vi "Encode.vi"(4 "Conf":T1, 5 "Controller 2 State":T2={"Left X"=0, "Left Y"=0, "Right X"=0, "Right Y"=0, "Button Encoding 9-12"=0, "Button Encoding 1-8"=0, "POV"=-1} {"POV" items=["None"=-1, "POV Up"=0, "POV Up Right"=1, "POV Right"=2, "POV Down Right"=3, "POV Down"=4, "POV Down Left"=5, "POV Left"=6, "POV Up Left"=7]}, 6 "Controller 1 State":T2={"Left X"=0, "Left Y"=0, "Right X"=0, "Right Y"=0, "Button Encoding 9-12"=0, "Button Encoding 1-8"=0, "POV"=-1} {"POV" items=["None"=-1, "POV Up"=0, "POV Up Right"=1, "POV Right"=2, "POV Down Right"=3, "POV Down"=4, "POV Down Left"=5, "POV Left"=6, "POV Up Left"=7]}) -> (0 "Joystick Data":string, 1 "Button Data":string)   [LabVIEW 2010, in "Packet Recorder.lvlib"]
uses:
  Packet Recorder.lvlib
  <vilib>/FTC/FTC ControllerState.ctl
  <vilib>/FTC/FTC POVState.ctl
  Components/Components.llb/Integer to Boolean Array_U16.vi
  Components/Components.lvlib
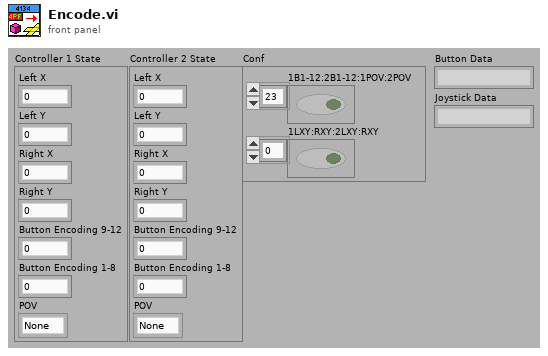
[diagram p1: front panel]
types:
  T1 = cluster{"1B1-12:2B1-12:1POV:2POV":bool[], "1LXY:RXY:2LXY:RXY":bool[]}
  T2 = typedef "FTC ControllerState.ctl" = cluster{"Left X":i8, "Left Y":i8, "Right X":i8, "Right Y":i8, "Button Encoding 9-12":u8, "Button Encoding 1-8":u8, "POV":T3}
  T3 = typedef "FTC POVState.ctl" = i8
  T4 = enum16{"big-endian, network order", "native, host order", "little-endian"}
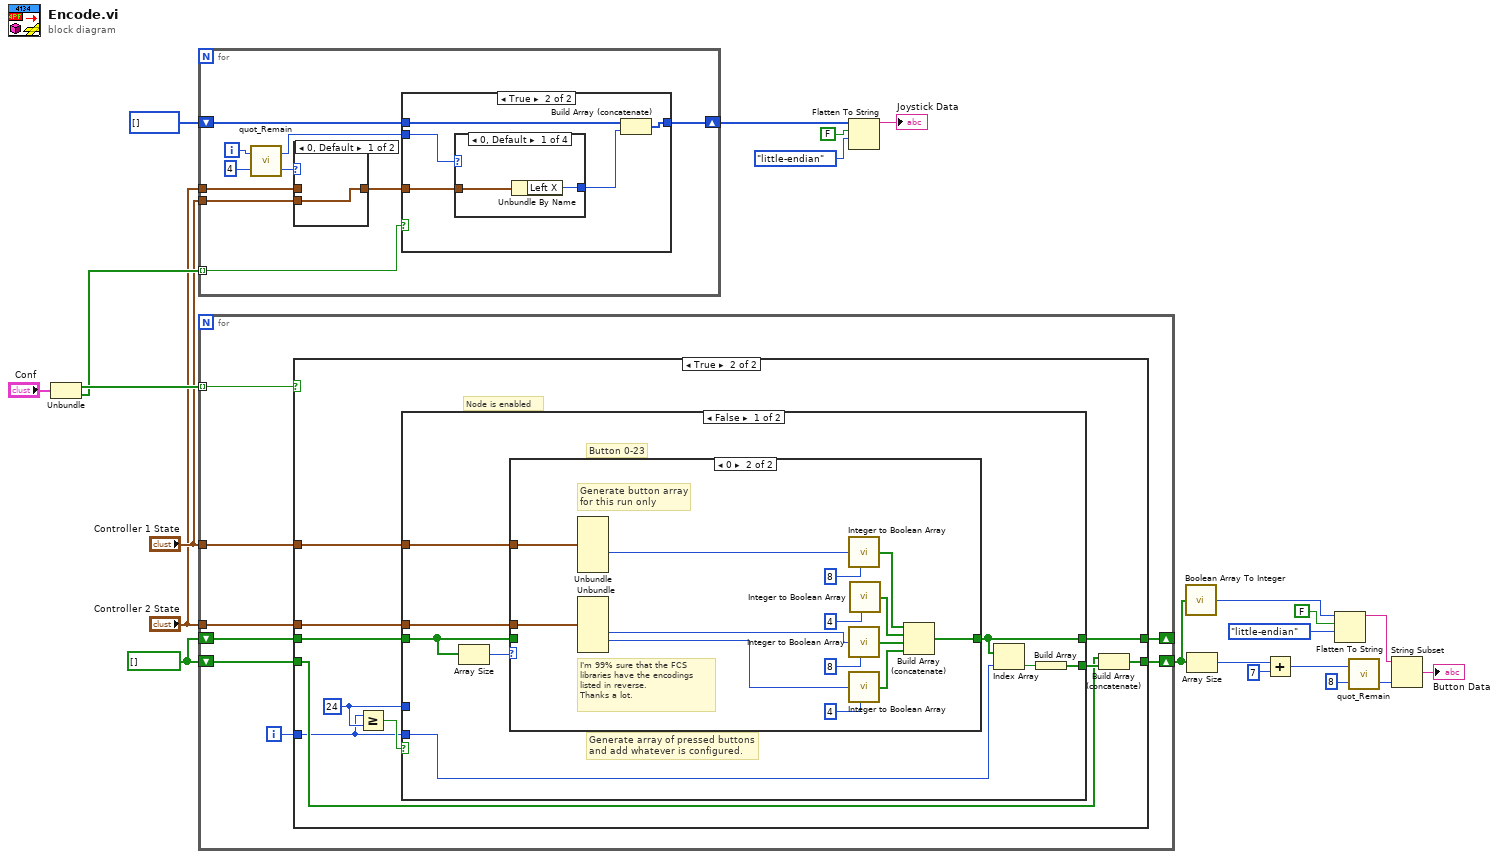
[diagram p0: block diagram]
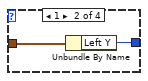
[diagram p4: hidden frame]
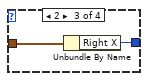
[diagram p5: hidden frame]
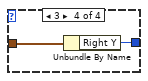
[diagram p6: hidden frame]
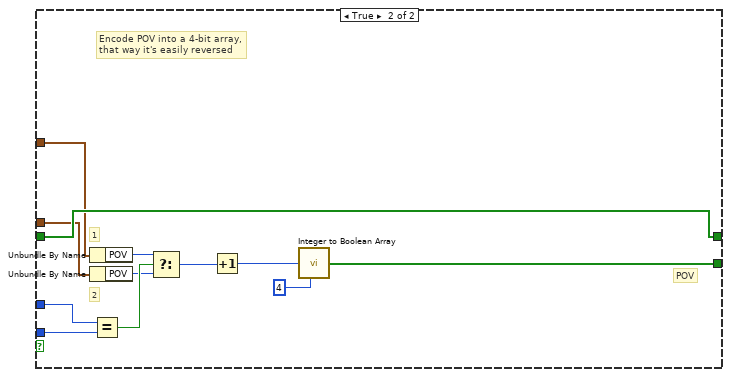
[diagram p9: hidden frame]
diagram:
  w20 = bool[] []
  n1 = Unbundle("Conf") -> ("1B1-12:2B1-12:1POV:2POV"=w22:bool[], "1LXY:RXY:2LXY:RXY"=w16:bool[])
  n2 = for {
    tunnel: w16 -> [w32] mode=indexing
    tunnel: "Controller 1 State" -> [w27]
    tunnel: "Controller 2 State" -> [w26]
    shift-right: [w24] -> w12
    shift-left: i8[] [] -> [w23]
    i -> [w31]
    n3 = call <vilib>:"quot_Remain.vi"("y"=4, "x"=w31) -> ("floor(x/y)"=w28:i32, "x-y*floor(x/y)"=w30:i32)
    n4 = case shown="0, Default" w28 {
      tunnel: w27 -> [w33 _]
      tunnel: w26 -> [_ w34]
      tunnel: [w33 w34] -> w25
      frame 0, Default {
      }
      frame 1 {
      }
    }
    n5 = case shown="True" w32 {
      tunnel: w30 -> [_ w40]
      tunnel: w25 -> [_ w39]
      tunnel: [w35 w37] -> w24
      tunnel: w23 -> [w35 w36]
      frame False {
      }
      frame True {
        n6 = case shown="0, Default" w40 {
          tunnel: [w42 w44 w45 w47] -> w38
          tunnel: w39 -> [w41 w43 w46 w48]
          frame 0, Default {
            n7 = Unbundle By Name(w41) -> ("Left X"=w42:i8)
          }
          frame 1 {
            n8 = Unbundle By Name(w43) -> ("Left Y"=w44:i8)
          }
          frame 2 {
            n9 = Unbundle By Name(w46) -> ("Right X"=w45:i8)
          }
          frame 3 {
            n10 = Unbundle By Name(w48) -> ("Right Y"=w47:i8)
          }
        }
        n11 = Build Array (concatenate)(w36, w38) -> (w37:i8[])
      }
    }
  }
  n12 = for {
    tunnel: w22 -> [w56] mode=indexing
    tunnel: "Controller 1 State" -> [w54]
    tunnel: "Controller 2 State" -> [w53]
    shift-right: [w52] -> w7
    shift-left: w20 -> [w51]
    shift-right: [w50] -> _
    shift-left: w20 -> [w49]
    i -> [w55]
    n13 = case shown="True" w56 {
      tunnel: w55 -> [_ w59]
      tunnel: w54 -> [_ w68]
      tunnel: w53 -> [_ w67]
      tunnel: [w58 w65] -> w52
      tunnel: w51 -> [w58 w64]
      tunnel: [w57 w63] -> w50
      tunnel: w49 -> [w57 w62]
      frame False {
        # "Node not enabled; maintain array state"
      }
      frame True {
        w60 = 24 ("y")
        # "Node is enabled"
        n14 = Greater Or Equal?(x=w59, y=w60) -> (x >= y?=w61:bool)
        n15 = case shown="False" w61 {
          tunnel: w68 -> [w76 w98]
          tunnel: w67 -> [w75 w97]
          tunnel: [w71 w93] -> w66
          tunnel: [w72 w103] -> w63
          tunnel: w62 -> [w74 w103]
          tunnel: w60 -> [_ w102]
          tunnel: w59 -> [w70 w101]
          frame False {
            # "Button 0-23"
            # "Generate array of pressed buttons\nand add whatever is configured."
            n16 = Array Size(array=w74) -> (size(s)=w73:i32)
            n17 = case shown="0" w73 {
              tunnel: w76 -> [_ w91]
              tunnel: w75 -> [_ w88]
              tunnel: [w77 w83] -> w72
              tunnel: w74 -> [w77 _]
              frame Default {
                # "Button array already generated"
              }
              frame 0 {
                # "I'm 99% sure that the FCS\nlibraries have the encodings\nlisted in reverse.\nThanks a lot."
                # "Generate button array\nfor this run only"
                n18 = Unbundle(w91) -> ("Button Encoding 9-12"=w80:u8)  [unwired: 6 out]
                n19 = Unbundle(w88) -> ("Button Encoding 9-12"=w79:u8, "Button Encoding 1-8"=w78:u8)  [unwired: 5 out]
                n20 = call-poly "Integer to Boolean Array.vi"("number"=w80, "minimum"=u32 8) -> ("Boolean array"=w81:bool[])  [unwired: 5 in]
                n21 = call-poly "Integer to Boolean Array.vi"("number"=w79, "minimum"=u32 8) -> ("Boolean array"=w85:bool[])  [unwired: 5 in]
                n22 = call-poly "Integer to Boolean Array.vi"("number"=w78, "minimum"=u32 4) -> ("Boolean array"=w84:bool[])  [unwired: 5 in]
                n23 = call-poly "Integer to Boolean Array.vi"("minimum"=u32 4) -> ("Boolean array"=w82:bool[])  [unwired: 6 in]
                n24 = Build Array (concatenate)(w81, w82, w85, w84) -> (w83:bool[])
              }
            }
            n25 = Index Array(array=w72, index=w70) -> (element=w69:bool)
            n26 = Build Array(w69) -> (w71:bool[])
          }
          frame True {
            # "Encode POV into a 4-bit array,\nthat way it's easily reversed"
            # "2"
            # "1"
            # "POV"
            n27 = Unbundle By Name(w98) -> ("POV"=w99:T3)
            n28 = Unbundle By Name(w97) -> ("POV"=w96:T3)
            n29 = Equal?(x=w102, y=w101) -> (x = y?=w100:bool)
            n30 = Select(t=w99, s=w100, f=w96) -> (s? t:f=w95:T3)
            n31 = Increment(x=w95) -> (x+1=w92:T3)
            n32 = call-poly "Integer to Boolean Array.vi"("number"=w92, "minimum"=u32 4) -> ("Boolean array"=w93:bool[])  [unwired: 5 in]
          }
        }
        n33 = Build Array (concatenate)(w64, w66) -> (w65:bool[])
      }
    }
  }
  n34 = Flatten To String(anything=w12, prepend array or string size? (T)=FALSE, byte order (0:big-endian, network order)=T4."little-endian") -> (data string=→"Joystick Data":string)  [unwired: 1 in, 2 out]
  n35 = call "Boolean Array To Integer.vi"("Boolean array"=w7) -> ("number"=w17:u32)  [unwired: 4 in]
  n36 = Array Size(array=w7) -> (size(s)=w6:i32)
  n37 = Add(x=w6, y=7) -> (x+y=w8:i32)
  n38 = Flatten To String(anything=w17, prepend array or string size? (T)=FALSE, byte order (0:big-endian, network order)=T4."little-endian") -> (data string=w3:string)  [unwired: 1 in, 2 out]
  n39 = call <vilib>:"quot_Remain.vi"("y"=8, "x"=w8) -> ("floor(x/y)"=w4:i32)  [unwired: 1 out]
  n40 = String Subset(string=w3, length (rest)=w4) -> (substring=→"Button Data":string)  [unwired: 1 in]
